vi "SwissSPAD Live_Download Single Image.vi"(4 "# 8-bit Images (1)":i32=1, 6 "Block Size":i32=-1, 8 "Error In":errorcluster, 9 "Discard First Image":bool=TRUE, 10 "Image":T1, 11 "Device Refnum":refnum<k24>) -> (0 "Error Out":errorcluster, 2 "Image Out":T1)   [LabVIEW 2021]
uses:
  D:/UCLA Thinkpad Google Drive/LabVIEW 2021 SP1/builds/SwissSPAD Live Distribution/Opal Kelly/C# Wrapper/v5.0.2/libFrontPanel-csharp.dll
  Opal Kelly/C# Wrapper/v5.0.2/libFrontPanel-csharp.dll
  <vilib>/vision/Image Controls.llb/IMAQ Image.ctl
  SwissSPAD Live_Settings List.ctl
  SwissSPAD Live_SS3 Displayed Image v2.ctl
  LV Tools/Logical Processors Used.vi
  Opal Kelly/C# Wrapper/okFrontPanelC#Wrapper.lvlib
  Variant/Variant to Data/Variant to Data.lvlib
panel:
  out "FPGA Error Out":errorcluster
  out "size(s)":i32
  out "CPU/Image":dbl
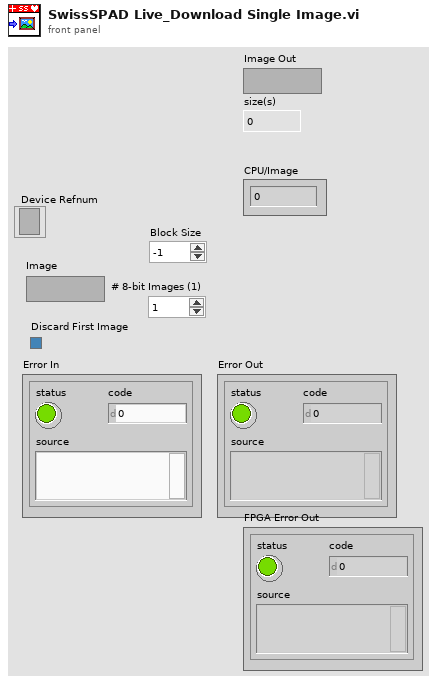
[diagram p1: front panel]
types:
  T1 = typedef "IMAQ Image.ctl" = refnum<image>
  T2 = typedef "SwissSPAD Live_Settings List.ctl" = enum16{"FPGA:Bottom Half", "FPGA:Top Half", "FPGA:Bottom Bitfile Path", "FPGA:Top Bitfile Path", "FPGA:Bottom Bitstream Version", "FPGA:Top Bitstream Version", "FPGA:Auto Reset FPGA", "FPGA:Bottom FPGA Serial Number", "FPGA:Top FPGA Serial Number", "FPGA:Detector PCB Version", "Acquisition Parameters:Microlens", "Acquisition Parameters:SS2 DAQ Parameters", "Acquisition Parameters:Gate Configuration Array", "Acquisition Parameters:SS3 DAQ Parameters", "Acquisition Parameters:Buffer Size (# 8-bit Gates)", "File Information:File Information", "File Information:# Datasets in Series", "File Information:Scrambled File Flag", "File Information:SS3 Gate Slip Correction", "File Information:SS3 Hot Pixel Mismatch Detection", "File Information:Delay between Datasets", "File Information:Save Sum of All Gates Preview", "Image Parameters:Image ROI Information", "Image Parameters:Image Binning Options", "Image Parameters:SS3 Displayed Image", "Image Parameters:Image Display Options", "Image Parameters:Use Histogram Cursors", "Image Parameter:FPGA Data to Display", "UI Settings:Histogram Bins Number", "UI Settings:Histogram Bin Size", "UI Settings:Use Image Display Options", "UI Settings:Verbose Settings", "UI Settings:Verbose Saving"}
  T3 = typedef "SwissSPAD Live_SS3 Displayed Image v2.ctl" = enum16{"G2 Gate", "INT Gate", "INT - G2"}
  T4 = typedef "SwissSPAD Live_Internal Variables.ctl" = cluster{"okCFrontPanelDevices Refnum":refnum<k24>, "Bottom Device Refnum":refnum<k24>, "Display Image":T1, "# Live Images":i32, "relative s":dbl, "# Image Sets":i32, "Message":string, "Current Image Set":i32, "# Datasets in Series":i32, "Current Dataset":i32, "Live Mode":bool, "Recording Mode":bool, "Record Button":refnum<vi>, "\nLive Button":refnum<vi>, "SwissSPAD Live Gate Image Data Q Name":string, "Discard First Image":bool, "Image Information":T5, "Image Binning Options":T6, "Bottom FPGA Serial Number":string, "Detector PCB Version":T7, "# Acquisitions":u32, "10 bits":bool, "Top FPGA Serial Number":string, "Top Device Refnum":refnum<k24>, "okCFrontPanel Refnum":refnum<k24>}
  T5 = typedef "SwissSPAD Live_Image ROI Information.ctl" = cluster{"Save ROI Only":bool, "Left":u16, "Top":u16, "Right":u16, "Bottom":u16, "Use Current ROI":bool}
  T6 = typedef "Image Binning Options.ctl" = cluster{"Use Image Binning":bool, "X Bin":i32, "Y Bin":i32}
  T7 = typedef "SwissSPAD Live_SSx PCB Version.ctl" = enum16{"unknown", "SS2 PCB1", "SS2 PCB2", "SS3 PCB1"}
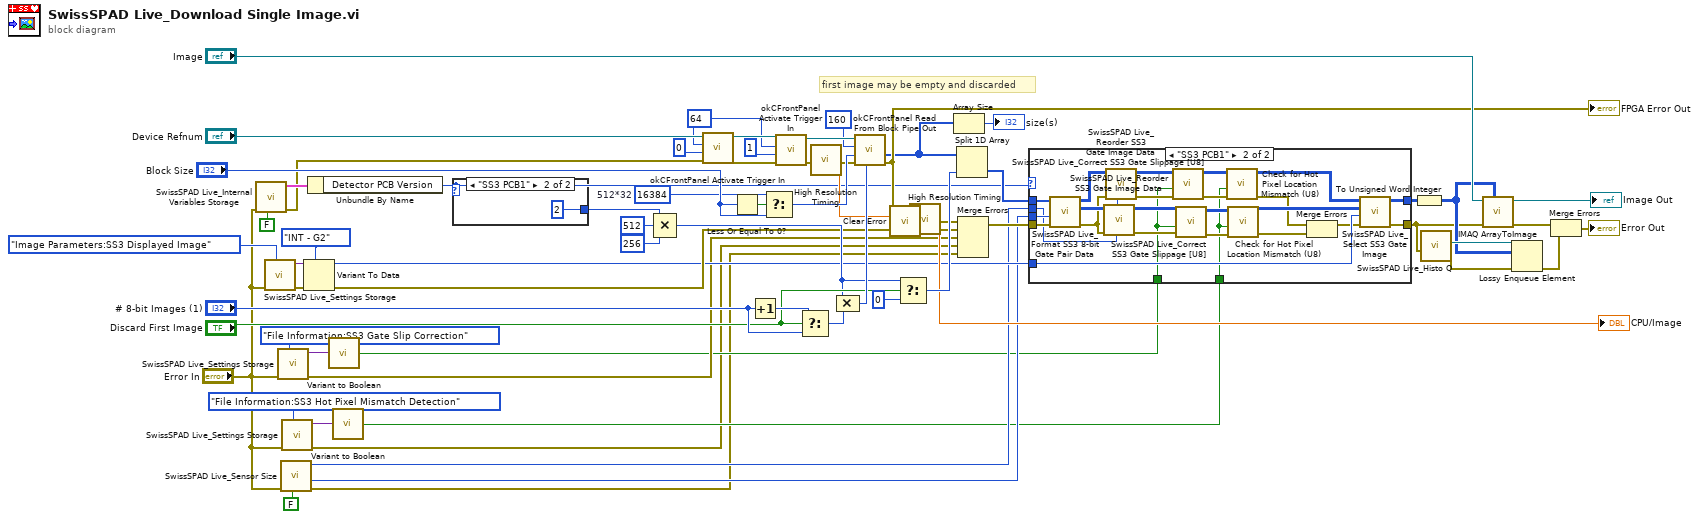
[diagram p0: block diagram]
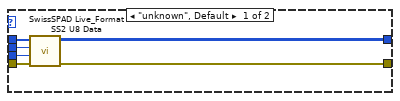
[diagram p2: hidden frame]
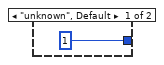
[diagram p3: hidden frame]
diagram:
  w16 = 16384  # 512*32
  w35 = 64 ("Endpoint Addr")
  # "first image may be empty and discarded"
  n1 = call "SwissSPAD Live_Internal Variables Storage.vi"("Set/Get(F)"=FALSE, "Error In"="Error In") -> ("Error Out"=w34:errorcluster, "SwissSPAD Live Internal Variables"=w36:T4)  [unwired: 8 in]
  n2 = call "SwissSPAD Live_Settings Storage.vi"("Settings List"=SwissSPAD_Live_Settings_List."Image Parameters:SS3 Displayed Image", "Error In"="Error In") -> ("Error Out"=w31:errorcluster, "Variant Data out"=w10:variant)  [unwired: 8 in]
  n3 = call "SwissSPAD Live_Settings Storage.vi"("Settings List"=SwissSPAD_Live_Settings_List."File Information:SS3 Gate Slip Correction", "Error In"="Error In") -> ("Error Out"=w12:errorcluster, "Variant Data out"=w7:variant)  [unwired: 8 in]
  n4 = call "SwissSPAD Live_Sensor Size.vi"("Set/Get(F)"=FALSE, "Error In"="Error In") -> ("Error Out"=w1:errorcluster, "Y size"=w20:i32, "X size"=w21:i32)  [unwired: 7 in]
  n5 = call "SwissSPAD Live_Settings Storage.vi"("Settings List"=SwissSPAD_Live_Settings_List."File Information:SS3 Hot Pixel Mismatch Detection", "Error In"="Error In") -> ("Error Out"=w2:errorcluster, "Variant Data out"=w6:variant)  [unwired: 8 in]
  n6 = Variant To Data(error in=w31, type=SwissSPAD_Live_SS3_Displayed_Image_v2."INT - G2" ("Image to Display"), Variant=w10) -> (data=w28:T3, error out=w30:errorcluster)
  n7 = Unbundle By Name(w36) -> ("Detector PCB Version"=w23:T7)
  n8 = call "Variant to Boolean.vi"("Variant"=w7) -> ("Value"=w11:bool)  [unwired: 8 in]
  n9 = call "Variant to Boolean.vi"("Variant"=w6) -> ("Value"=w5:bool)  [unwired: 8 in]
  n10 = case shown="\"SS3 PCB1\"" w23 {
    tunnel: [1 2] -> w33
    frame "unknown", Default {
    }
    frame "SS3 PCB1" {
    }
  }
  n11 = Compound Arithmetic op=MULTIPLY(w33, 512 ("value"), 256 ("value")) -> (w45:i32)
  n12 = call "okCFrontPanel Activate Trigger In.vi"("Error In"=w34, "Bit"=0, "Endpoint Addr"=w35, "okCFrontPanel Refnum"="Device Refnum") -> ("Error Out"=w66:errorcluster, "okCFrontPanel Refnum"=w65:refnum<k24>)  [unwired: 6 in]
  n13 = Less Or Equal To 0?(x="Block Size") -> (x <= 0?=w58:bool)
  n14 = Increment(x="# 8-bit Images (1)") -> (x+1=w48:i32)
  n15 = Select(t=w16, s=w58, f="Block Size") -> (s? t:f=w57:i32)
  n16 = call "okCFrontPanel Activate Trigger In.vi"("Error In"=w66, "Bit"=1, "Endpoint Addr"=w35, "okCFrontPanel Refnum"=w65) -> ("Error Out"=w42:errorcluster, "okCFrontPanel Refnum"=w62:refnum<k24>)  [unwired: 6 in]
  n17 = Select(t=w48, s="Discard First Image", f="# 8-bit Images (1)") -> (s? t:f=w47:i32)
  n18 = call "High Resolution Timing.vi"("Error In"=w42) -> ("elapsed (relative) seconds"=w39:dbl, "Error Out"=w41:errorcluster)  [unwired: 16 in, 1 out]
  n19 = Compound Arithmetic op=MULTIPLY(w45, w47) -> (w54:i32)
  n20 = call "okCFrontPanel Read From Block Pipe Out.vi"("Length"=w54, "Error In"=w41, "Block Size"=w57, "Endpoint Addr"=160, "okCFrontPanel Refnum"=w62) -> ("Error Out"=w26:errorcluster, "BYTEARRAY"=w25:u8[])  [unwired: 4 in, 1 out]
  "FPGA Error Out" <- w26
  n21 = call "Clear Error.vi"("Error In"=w26) -> ("no Error Out"=w22:errorcluster)  [unwired: 8 in]
  n22 = Select(t=w45, s="Discard First Image", f=0) -> (s? t:f=w43:i32)
  n23 = call "High Resolution Timing.vi"("relative seconds (NaN)"=w39, "Error In"=w22) -> ("elapsed (relative) seconds"=→"CPU/Image":dbl, "Error Out"=w40:errorcluster)  [unwired: 15 in, 1 out]
  n24 = Array Size(array=w25) -> (size(s)=→"size(s)":i32)
  n25 = Split 1D Array(array=w25, index=w43) -> (second subarray=w55:u8[])  [unwired: 1 out]
  n26 = Merge Errors(w40, w30, w12, w2, w1) -> (w32:errorcluster)
  n27 = case shown="\"SS3 PCB1\"" w23 {
    tunnel: w55 -> [w75 w99]
    tunnel: w32 -> [w74 w100]
    tunnel: [w73 w97] -> w13
    tunnel: [w72 w96] -> w15
    tunnel: w20 -> [w71 w98]
    tunnel: w21 -> [w70 w93]
    tunnel: w28 -> [_ w95]
    tunnel: w11 -> [_ w83]
    tunnel: w5 -> [_ w76]
    frame "unknown", Default {
      n28 = call "SwissSPAD Live_Format SS2 U8 Data.vi"("Error In"=w74, "Y Resolution"=w71, "X Resolution"=w70, "Flattened Image"=w75) -> ("Error Out"=w73:errorcluster, "Image out"=w72:u8[][])  [unwired: 6 in]
    }
    frame "SS3 PCB1" {
      n29 = call "SwissSPAD Live_Format SS3 8-bit Gate Pair Data.vi"("Error In"=w100, "Y Resolution (250)"=w98, "Flattened Image (512x256x2)"=w99) -> ("Error Out"=w91:errorcluster, "Gate 2 (512x250)"=w92:u8[][], "Integral Gate (512x250)"=w94:u8[][])  [unwired: 6 in]
      n30 = call "SwissSPAD Live_Reorder SS3 Gate Image Data.vi"("X Resolution (500)"=w93, "Error In"=w91, "Interlaced Gate (512x250)"=w92) -> ("Error Out"=w86:errorcluster, "De-interlaced Gate (500x250)"=w87:u8[][])  [unwired: 7 in]
      n31 = call "SwissSPAD Live_Reorder SS3 Gate Image Data.vi"("X Resolution (500)"=w93, "Error In"=w91, "Interlaced Gate (512x250)"=w94) -> ("Error Out"=w88:errorcluster, "De-interlaced Gate (500x250)"=w89:u8[][])  [unwired: 7 in]
      n32 = call "SwissSPAD Live_Correct SS3 Gate Slippage [U8].vi"("Error In"=w88, "Slippage Correction (T)"=w83, "Array in"=w89) -> ("Error Out"=w79:errorcluster, "Array out"=w80:u8[][])  [unwired: 6 in, 1 out]
      n33 = call "SwissSPAD Live_Correct SS3 Gate Slippage [U8].vi"("Error In"=w86, "Slippage Correction (T)"=w83, "Array in"=w87) -> ("Error Out"=w84:errorcluster, "Array out"=w85:u8[][])  [unwired: 6 in, 1 out]
      n34 = call "Check for Hot Pixel Location Mismatch (U8).vi"("error in (no error)"=w79, "SS3 Hot Pixel Mismatch Detection"=w76, "Array in"=w80) -> ("error out"=w77:errorcluster, "Array (dup)"=w78:u8[][])  [unwired: 7 in]
      n35 = call "Check for Hot Pixel Location Mismatch (U8).vi"("error in (no error)"=w84, "SS3 Hot Pixel Mismatch Detection"=w76, "Array in"=w85) -> ("error out"=w81:errorcluster, "Array (dup)"=w82:u8[][])  [unwired: 7 in]
      n36 = Merge Errors(w77, w81) -> (w90:errorcluster)
      n37 = call "SwissSPAD Live_Select SS3 Gate Image.vi"("Error In"=w90, "Image to Display"=w95, "Gate 2 (500x250)"=w82, "INT Gate (500x250)"=w78) -> ("Error Out"=w97:errorcluster, "Selected Gate (500x250)"=w96:u8[][])  [unwired: 5 in, 1 out]
    }
  }
  n38 = To Unsigned Word Integer(number=w15) -> (unsigned 16bit integer=w14:u16[][])
  n39 = call "SwissSPAD Live_Histo Q.vi"("error in (no error)"=w13) -> ("error out"=w50:errorcluster, "SS2 Live Histo Q"=w53:refnum<queue>)  [unwired: 5 in]
  n40 = call "IMAQ ArrayToImage"("Image Pixels (U16)"=w14, "error in (no error)"=w13, "Image"="Image") -> ("error out"=w59:errorcluster, "Image Out"=→"Image Out":T1)  [unwired: 7 in]
  n41 = Lossy Enqueue Element(queue=w53, element=w14, error in (no error)=w50) -> (error out=w51:errorcluster)  [unwired: 3 out]
  n42 = Merge Errors(w59, w51) -> (→"Error Out":errorcluster)
